vi "StartingLocations.vi"(11 "Index":i32) -> (3 "Location":cluster{dbl, dbl})   [LabVIEW 2018]
uses:
  Robot-Project/Configuration/Constants.vi
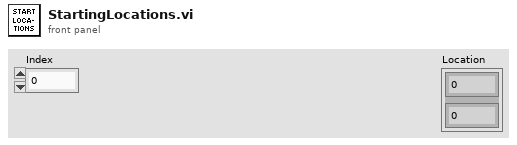
[diagram p1: front panel]
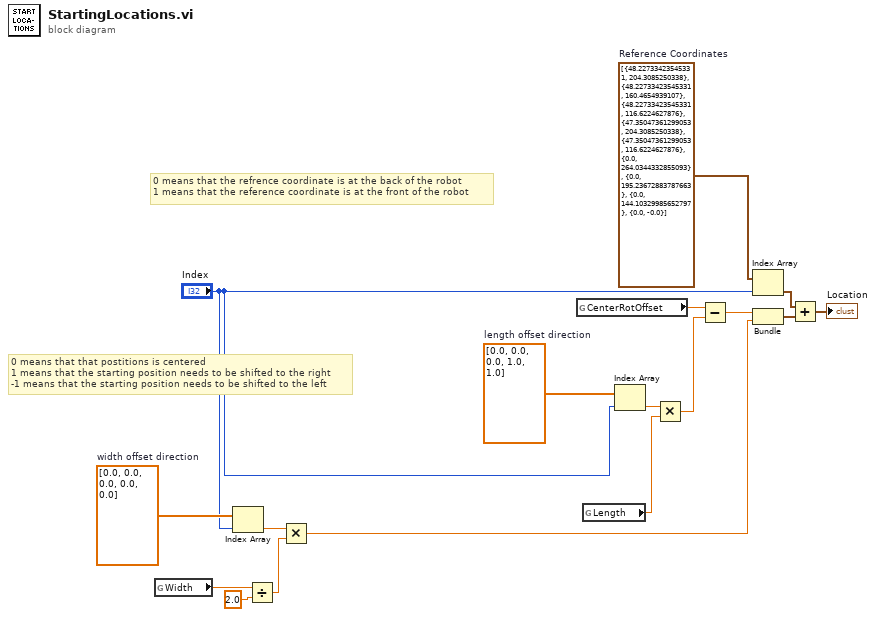
[diagram p0: block diagram]
diagram:
  w5 = dbl[] [0.0, 0.0, 0.0, 1.0, 1.0]  # length offset direction
  w12 = dbl[] [0.0, 0.0, 0.0, 0.0, 0.0]  # width offset direction
  w13 = cluster{dbl, dbl}[] [{48.22733423545331, 204.3085250338}, {48.22733423545331, 160.4654939107}, {48.22733423545331, 116.6224627876}, {47.35047361299053, 204.3085250338}, {47.35047361299053, 116.6224627876}, {0.0, 264.0344332855093}, {0.0, 195.23672883787663}, {0.0, 144.10329985652797}, {0.0, -0.0}]  # Reference Coordinates
  # "0 means that that postitions is centered\n1 means that the starting position needs to be shifted to the right\n-1 means that the starting position needs to be shifted to the left"
  # "0 means that the refrence coordinate is at the back of the robot\n1 means that the reference coordinate is at the front of the robot"
  n1 = global read "Constants.vi" "Width"() -> (w10:dbl)
  n2 = Index Array(array=w12, index="Index") -> (element=w15:dbl)
  n3 = Divide(x=w10, y=2.0) -> (x/y=w11:dbl)
  n4 = Multiply(x=w15, y=w11) -> (x*y=w16:dbl)
  n5 = global read "Constants.vi" "CenterRotOffset"() -> (w6:dbl)
  n6 = global read "Constants.vi" "Length"() -> (w7:dbl)
  n7 = Index Array(array=w5, index="Index") -> (element=w4:dbl)
  n8 = Multiply(x=w4, y=w7) -> (x*y=w2:dbl)
  n9 = Subtract(x=w6, y=w2) -> (x-y=w1:dbl)
  n10 = Index Array(array=w13, index="Index") -> (element=w14:cluster{dbl, dbl})
  n11 = Bundle(w1, w16) -> (w17:cluster{dbl, dbl})  [unwired: 1 in]
  n12 = Add(x=w14, y=w17) -> (x+y=→"Location":cluster{dbl, dbl})
